vi "Condition Msg Output Output VI.vi"(8 "error in":errorcluster, 9 "Conn Pane Terminals.Msg Output Indicator":i32[](array[numeric]), 10 "Name Msg Output Refs.Output VI":refnum<vi>) -> (0 "error out":errorcluster)   [LabVIEW 2025, in "_Msg Rescript.lvlib" / "_Msg Rescript.lvclass"]
uses:
  _Msg Rescript.lvclass
  _Msg Rescript.lvclass/_Msg Rescript.ctl
  <vilib>/Utility/traverseref.llb/TRef TravTarget.ctl
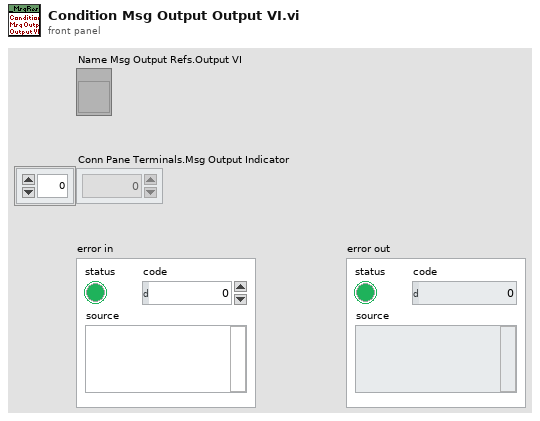
[diagram p1: front panel]
types:
  T1 = typedef "TRef TravTarget.ctl" = enum16{"FP", "BD", "Other"}
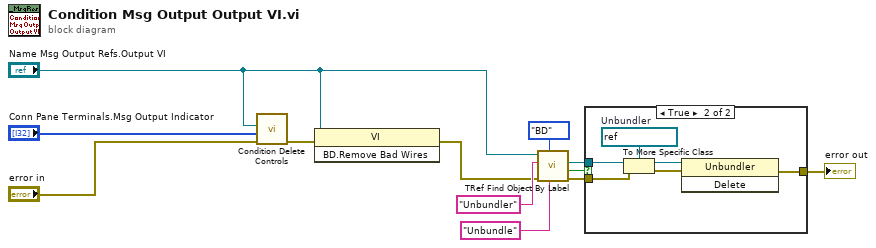
[diagram p0: block diagram]
diagram:
  n1 = call "Condition Delete Controls.vi"("error in"="error in", "Control Terminals"="Conn Pane Terminals.Msg Output Indicator", "VI Ref"="Name Msg Output Refs.Output VI") -> ("error out"=w11:errorcluster)  [unwired: 8 in]
  n2 = invoke class="VI" method="BD.Remove Bad Wires"(reference="Name Msg Output Refs.Output VI", error in=w11) -> (error out=w5:errorcluster)  [unwired: 1 in, 2 out]
  n3 = call <vilib>:"TRef Find Object By Label.vi"("Label"="Unbundle", "Traverse Target"=TRef_TravTarget."BD", "error in (no error)"=w5, "Class Name"="Unbundler", "VI Ref"="Name Msg Output Refs.Output VI") -> ("error out"=w10:errorcluster, "Found?"=w3:bool, "Found Obj Ref"=w9:refnum<vi>)  [unwired: 3 in, 1 out]
  n4 = case shown="True" w3 {
    tunnel: w10 -> [w13 w19]
    tunnel: w9 -> [_ w17]
    tunnel: [w13 w15] -> w4
    frame False {
    }
    frame True {
      w18 = refnum<vi> refnum  # Unbundler
      n5 = To More Specific Class(target class=w18, reference=w17, error in=w19) -> (specific class reference=w16:refnum<vi>, error out=w14:errorcluster)
      n6 = invoke class="Unbundler" method="Delete"(reference=w16, error in=w14) -> (error out=w15:errorcluster)  [unwired: 1 in, 2 out]
    }
  }
  "error out" <- w4
